vi "Lambda_Configuration_ex_versao2.vi"() -> ()   [LabVIEW 2015]
uses:
  <vilib>/Utility/error.llb/DialogType.ctl
  <vilib>/Utility/file.llb/Read From Spreadsheet File (DBL).vi
  <vilib>/Utility/NIReport.llb/NI_report.lvclass
  <vilib>/addons/_office/NI_ReportGenerationToolkit.lvlib
panel:
  in  "LED Measurement":dbl
  out "error out":errorcluster
  in  "report file path":path=path "C:/Users/Tulio/Documents/Testes/Backup excel/backup excel.xlsx"
  out "Voltage":dbl[](graph)
  out "Current":dbl[](graph)
  in  "Load File?":bool
  in  "?":bool
  out "Output Current":dbl format="%.6f"
  out "Output Voltage":dbl format="%.6f"
  out "Serial Number:":string
  out "error?":bool
  out "Model:":string
  in  "Reset (T)":bool=TRUE
  in  "BAUD":u16(ring)=3 items=["1200", "2400", "4800", "9600", "19200"]
  in  "GEN Addr":i16=6
  in  "VISA name":refnum<visa-resource-name>
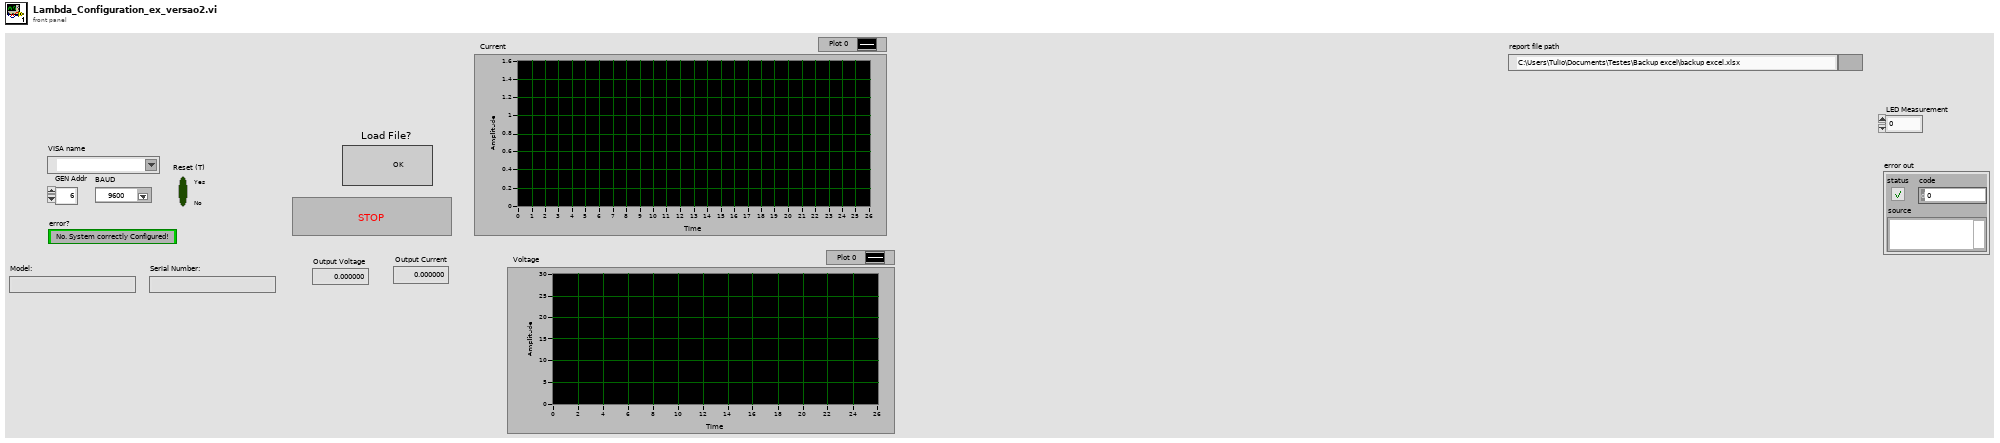
[diagram p1: front panel]
types:
  T1 = enum16{"Standard Report", "HTML", "Word", "Excel"}
  T2 = typedef "DialogType.ctl" = u16
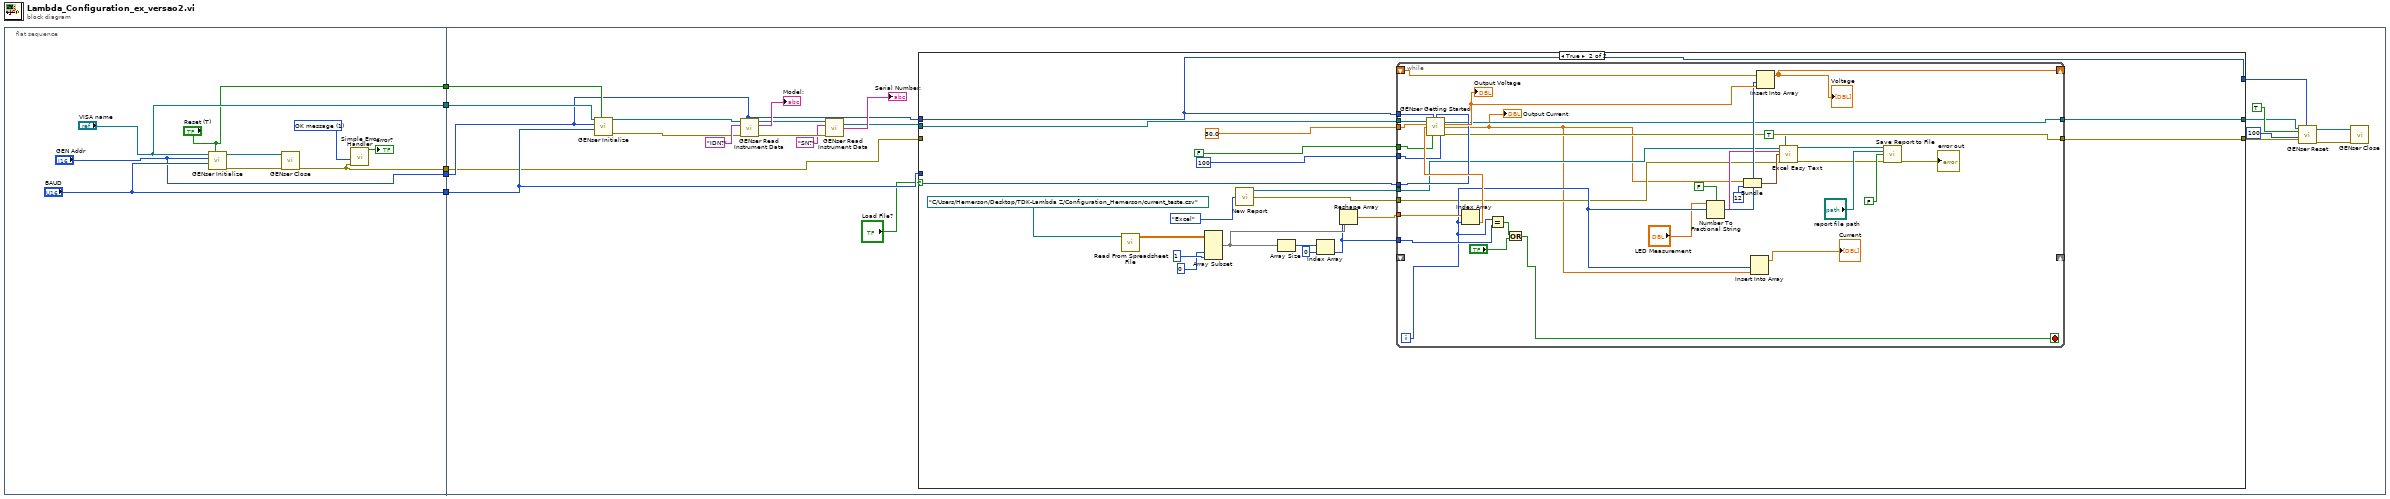
[diagram p0: block diagram]
diagram:
  n1 = flat-sequence {
    tunnel: ["BAUD"] -> w5
    tunnel: ["GEN Addr"] -> w4
    tunnel: ["VISA name"] -> w3
    tunnel: ["Reset (T)"] -> w2
    tunnel: [w6] -> w1
    tunnel: w5 -> [w20]
    tunnel: w4 -> [w22]
    tunnel: w3 -> [w29]
    tunnel: w2 -> [w30]
    tunnel: w1 -> [w15]
    frame #0 {
      w12 = T2 1 items=["no dialog", "OK message", "continue or stop message", "OK message + warnings", "continue/stop + warnings"] ("type of dialog (OK msg:1)")
      n2 = call "GENser Initialize.vi"("Reset (T)"="Reset (T)", "BAUD"="BAUD", "GEN Addr"="GEN Addr", "VISA name"="VISA name") -> ("error out"=w13:errorcluster, "VISA out"=w14:refnum<visa-resource-name>)  [unwired: 6 in]
      n3 = call "GENser Close.vi"("error"=w13, "VISA name"=w14) -> ("error out"=w6:errorcluster)  [unwired: 9 in]
      n4 = call <vilib>:"Simple Error Handler.vi"("type of dialog (OK msg:1)"=w12, "error in (no error)"=w6) -> ("error?"=→"error?":bool)  [unwired: 3 in, 4 out]
    }
    frame #1 {
      n5 = call "GENser Initialize.vi"("Reset (T)"=w30, "BAUD"=w20, "GEN Addr"=w22, "VISA name"=w29) -> ("error out"=w27:errorcluster, "VISA out"=w28:refnum<visa-resource-name>)  [unwired: 6 in]
      n6 = call "GENser Read Instrument Data.vi"("GEN Addr"=w22, "error"=w27, "Query"="IDN?", "VISA"=w28) -> ("error out"=w33:errorcluster, "Response"=→"Model:":string, "VISA out"=w34:refnum<visa-resource-name>)  [unwired: 4 in, 1 out]
      n7 = call "GENser Read Instrument Data.vi"("error"=w33, "Query"="SN?", "VISA"=w34) -> ("Response"=→"Serial Number:":string, "VISA out"=w21:refnum<visa-resource-name>)  [unwired: 5 in, 2 out]
      n8 = case shown="True" "Load File?" {
        tunnel: w22 -> [w39 w48]
        tunnel: w21 -> [w38 w49]
        tunnel: w20 -> [_ w52]
        tunnel: [w37 w44] -> w19
        tunnel: [w38 w43] -> w18
        tunnel: [w39 w48] -> w17
        tunnel: w15 -> [w37 _]
        frame False {
        }
        frame True {
          n9 = call-poly <vilib>:"Read From Spreadsheet File.vi"("file path (dialog if empty)"=path "C:/Users/Hemerson/Desktop/TDK-Lambda Z/Configuration_Hemerson/current_teste.csv") -> ("all rows"=w54:dbl[][])  [unwired: 6 in, 4 out]
          n10 = Array Subset "Array Subset"(array=w54, index (col)=0 ("index"), length (col)=1 ("length")) -> (w56:dbl[][])  [unwired: 2 in]
          n11 = call <vilib>:"New Report.vi"("report type"=T1."Excel") -> ("report out"=w41:refnum<class "NI_report.lvclass">, "error out"=w40:errorcluster)  [unwired: 13 in]
          n12 = Array Size(array=w56) -> (size(s)=w57:i32[])
          n13 = Index Array "Index Array"(array=w57, index=0) -> (element=w45:i32)
          n14 = Reshape Array "Reshape Array"(w56, w45) -> (w46:dbl[])
          n15 = while {
            shift-right: _ -> [_]
            shift-left: _ -> [_]
            tunnel: w52 -> [w87]
            tunnel: u32 100 ("Settle (0 mS)") -> [w86]
            tunnel: FALSE ("Reset (T)") -> [w85]
            tunnel: w49 -> [w84]
            tunnel: w48 -> [w83]
            tunnel: 30.0 ("Voltage Limit") -> [w82]
            tunnel: w46 -> [w81]
            tunnel: w45 -> [w80]
            shift-right: [w79] -> _
            shift-left: _ -> [w78]
            tunnel: [w76] -> w44
            tunnel: [w75] -> w43
            tunnel: w41 -> [w62]
            tunnel: w40 -> [w61]
            i -> [w77]
            stop <- w74 stop-if-true
            n16 = Index Array(array=w81, index=w77) -> (element=w89:dbl)
            n17 = call "GENser Getting Started.vi"("VISA"=w84, "GEN Addr"=w83, "BAUD"=w87, "Voltage Limit"=w82, "Current Limit"=w89, "Reset (T)"=w85, "Settle (0 mS)"=w86) -> ("VISA out"=w75:refnum<visa-resource-name>, "Output Voltage"=w92:dbl, "Output Current"=w60:dbl, "error out"=w76:errorcluster)  [unwired: 5 in]
            "Output Current" <- w60
            "Output Voltage" <- w92
            n18 = Equal?(x=w77, y=w80) -> (x = y?=w90:bool)
            n19 = Or(x=w90, y="?") -> (x .or. y?=w74:bool)
            n20 = Number To Fractional String(use system decimal point (T)=FALSE, number="LED Measurement") -> (F-format string=w63:string)  [unwired: 2 in]
            n21 = Bundle("Output Current"=w60, "offset (0)"=12) -> (w68:cluster{"Output Current":dbl, "offset (0)":i32})  [unwired: 1 in]
            n22 = Insert Into Array(index=w77, new element=w60) -> (→"Current":dbl[])  [unwired: 1 in]
            n23 = Insert Into Array(array=w78, index=w77, new element=w92) -> (w79:dbl[])
            "Voltage" <- w79
            n24 = call <vilib>:"Excel Easy Text.vi"("report in"=w62, "border? (F)"=TRUE, "text"=w63, "start (-1, -1)"=w68, "error in (no error)"=w61) -> ("report out"=w65:refnum<class "NI_report.lvclass">, "error out"=w66:errorcluster)  [unwired: 6 in, 3 out]
            n25 = call-dynamic "Save Report to File.vi"("report in"=w65, "report file path"="report file path", "prompt to replace? (F)"=FALSE, "error in (no error)"=w66) -> ("error out"=→"error out":errorcluster)  [unwired: 10 in, 1 out]
          }
        }
      }
      n26 = call "GENser Reset.vi"("GEN Addr"=w17, "error"=w19, "Settle (0 mS)"=u32 100, "Reset (T)"=TRUE, "VISA"=w18) -> ("error out"=w23:errorcluster, "VISA out"=w25:refnum<visa-resource-name>)  [unwired: 5 in]
      n27 = call "GENser Close.vi"("error"=w23, "VISA name"=w25) -> ()  [unwired: 9 in, 1 out]
    }
  }
